vi "XYpos.vi"() -> ()   [LabVIEW 2010]
uses:
  <vilib>/DAQmx/write.llb/DAQmx Write (Digital Bool 1Line 1Point).vi
  <vilib>/DAQmx/read.llb/DAQmx Read (Analog DBL 1Chan 1Samp).vi
  <vilib>/DAQmx/write.llb/DAQmx Write (Analog DBL 1Chan 1Samp).vi
  <vilib>/DAQmx/create/channels.llb/DAQmx Create Channel (AO-Voltage-Basic).vi
  <vilib>/DAQmx/create/channels.llb/DAQmx Create Channel (DO-Digital Output).vi
  <vilib>/daqmx/miscellaneous.llb/DAQmx Fill In Error Info.vi
  <vilib>/DAQmx/create/channels.llb/DAQmx Create Channel (AI-Voltage-Basic).vi
panel:
  out "data 3":dbl format="%0.2f"
  in  "data":bool
  in  "Y":dbl format="%0.2f"
  in  "X":dbl format="%0.2f"
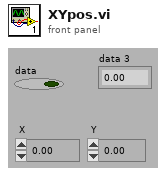
[diagram p1: front panel]
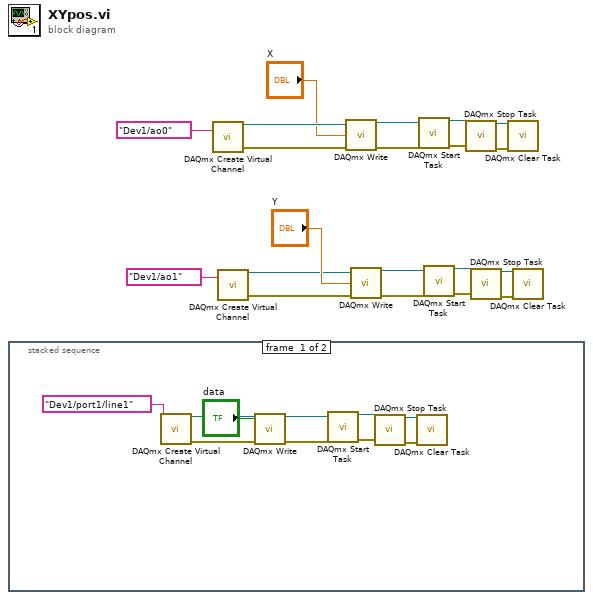
[diagram p0: block diagram]
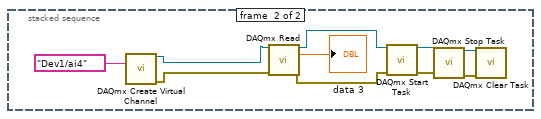
[diagram p2: hidden frame]
diagram:
  n1 = stacked-sequence {
    frame #0 {
      n2 = call-poly <vilib>:"DAQmx Create Virtual Channel.vi"("lines"=tag "Dev1/port1/line1") -> ("task out"=w23:refnum<k21>, "error out"=w21:errorcluster)  [unwired: 13 in]
      n3 = call-poly <vilib>:"DAQmx Write.vi"("task/channels in"=w23, "data"="data", "error in"=w21) -> ("task out"=w24:refnum<k21>, "error out"=w25:errorcluster)  [unwired: 10 in, 1 out]
      n4 = call <vilib>:"DAQmx Start Task.vi"("task/channels in"=w24, "error in"=w25) -> ("task out"=w26:refnum<k21>, "error out"=w27:errorcluster)  [unwired: 12 in]
      n5 = call <vilib>:"DAQmx Stop Task.vi"("task/channels in"=w26, "error in"=w27) -> ("task out"=w28:refnum<k21>, "error out"=w29:errorcluster)  [unwired: 12 in]
      n6 = call <vilib>:"DAQmx Clear Task.vi"("task in"=w28, "error in"=w29) -> ()  [unwired: 13 in, 1 out]
    }
    frame #1 {
      n7 = call-poly <vilib>:"DAQmx Create Virtual Channel.vi"("physical channels"=tag "Dev1/ai4") -> ("task out"=w39:refnum<k21>, "error out"=w31:errorcluster)  [unwired: 13 in]
      n8 = call-poly <vilib>:"DAQmx Read.vi"("task/channels in"=w39, "error in"=w31) -> ("task out"=w33:refnum<k21>, "data"=→"data 3":dbl, "error out"=w32:errorcluster)  [unwired: 11 in]
      n9 = call <vilib>:"DAQmx Start Task.vi"("task/channels in"=w33, "error in"=w32) -> ("task out"=w37:refnum<k21>, "error out"=w36:errorcluster)  [unwired: 12 in]
      n10 = call <vilib>:"DAQmx Stop Task.vi"("task/channels in"=w37, "error in"=w36) -> ("task out"=w35:refnum<k21>, "error out"=w34:errorcluster)  [unwired: 12 in]
      n11 = call <vilib>:"DAQmx Clear Task.vi"("task in"=w35, "error in"=w34) -> ()  [unwired: 13 in, 1 out]
    }
  }
  n12 = call-poly <vilib>:"DAQmx Create Virtual Channel.vi"("physical channels"=tag "Dev1/ao0") -> ("task out"=w20:refnum<k21>, "error out"=w16:errorcluster)  [unwired: 13 in]
  n13 = call-poly <vilib>:"DAQmx Create Virtual Channel.vi"("physical channels"=tag "Dev1/ao1") -> ("task out"=w3:refnum<k21>, "error out"=w7:errorcluster)  [unwired: 13 in]
  n14 = call-poly <vilib>:"DAQmx Write.vi"("task/channels in"=w20, "data"="X", "error in"=w16) -> ("task out"=w18:refnum<k21>, "error out"=w17:errorcluster)  [unwired: 10 in, 1 out]
  n15 = call-poly <vilib>:"DAQmx Write.vi"("task/channels in"=w3, "data"="Y", "error in"=w7) -> ("task out"=w5:refnum<k21>, "error out"=w6:errorcluster)  [unwired: 10 in, 1 out]
  n16 = call <vilib>:"DAQmx Start Task.vi"("task/channels in"=w18, "error in"=w17) -> ("task out"=w15:refnum<k21>, "error out"=w14:errorcluster)  [unwired: 12 in]
  n17 = call <vilib>:"DAQmx Start Task.vi"("task/channels in"=w5, "error in"=w6) -> ("task out"=w8:refnum<k21>, "error out"=w9:errorcluster)  [unwired: 12 in]
  n18 = call <vilib>:"DAQmx Stop Task.vi"("task/channels in"=w15, "error in"=w14) -> ("task out"=w13:refnum<k21>, "error out"=w12:errorcluster)  [unwired: 12 in]
  n19 = call <vilib>:"DAQmx Stop Task.vi"("task/channels in"=w8, "error in"=w9) -> ("task out"=w10:refnum<k21>, "error out"=w11:errorcluster)  [unwired: 12 in]
  n20 = call <vilib>:"DAQmx Clear Task.vi"("task in"=w13, "error in"=w12) -> ()  [unwired: 13 in, 1 out]
  n21 = call <vilib>:"DAQmx Clear Task.vi"("task in"=w10, "error in"=w11) -> ()  [unwired: 13 in, 1 out]
